vi "Write Startup Launch Nested Views Msg.vi"(8 "error in (no error)":errorcluster, 10 "Launch Nested Views Msg":refnum<class "Launch Nested Views Msg.lvclass">, 11 "IViewManager in":refnum<class "IViewManager.lvclass">) -> (0 "error out":errorcluster, 3 "IViewManager out":refnum<class "IViewManager.lvclass">)   [LabVIEW 2015, in "IViewManager.lvlib" / "IViewManager.lvclass"]
doc: "<License>\nCopyright © 2017 Composed Systems, LLC | All rights reserved\nwww.composed.io\n\nAuthor: Ethan Stern <ethan.stern@composed.io>\n\nThis software is provided \"AS IS\" WITHOUT WARRANTIES, either express or implied, AND IS FOR EDUCATIONAL PURPOSES ONLY.\n</License>"
uses:
  IViewManager.lvclass
  IViewManager Messages/Launch Nested Views Msg/Launch Nested Views Msg.lvclass
  IViewManager.lvclass/IViewManager.ctl
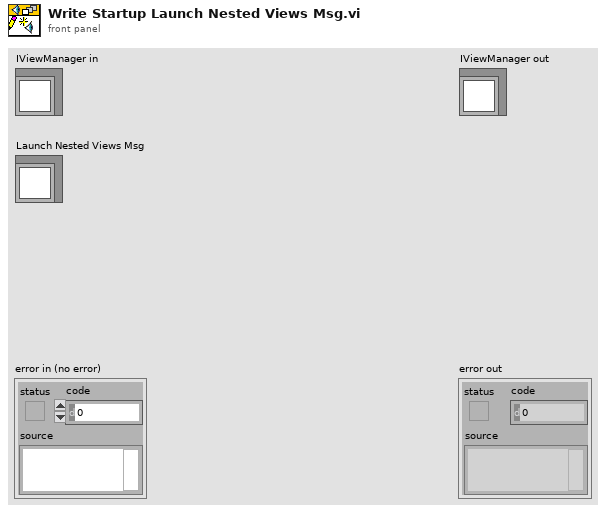
[diagram p1: front panel]
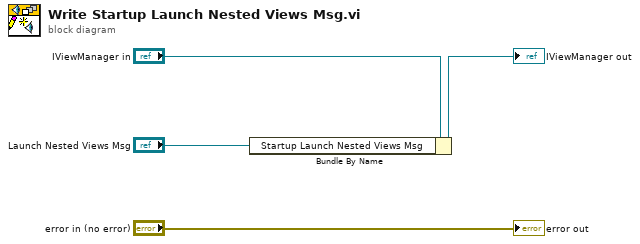
[diagram p0: block diagram]
diagram:
  n1 = Bundle By Name(cluster="IViewManager in", "Startup Launch Nested Views Msg"="Launch Nested Views Msg") -> (→"IViewManager out":refnum<class "IViewManager.lvclass">)
  "error out" <- "error in (no error)"
